vi "Auto Ground Manipulator Command_wrapper.vi"() -> ()   [LabVIEW 2020]
uses:
  <vilib>/Rock Robotics/WPI/Framework/Command Status Info.ctl
  <vilib>/Rock Robotics/WPI/Framework/Completion Status.ctl
  <vilib>/Rock Robotics/WPI/Framework/Completion Notifier.ctl
  intake sub/Implementation/Typedef/intake typedef.ctl
panel:
  out "Command Info Out":T1
  in  "intake modes":T4
  in  "Command Info In":T1
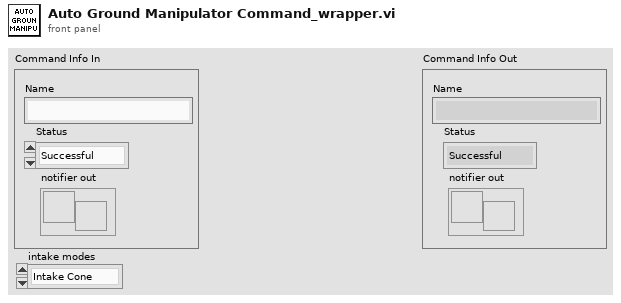
[diagram p1: front panel]
types:
  T1 = typedef "Command Status Info.ctl" = cluster{"Name":string, "Status":T2, "notifier out":T3}
  T2 = typedef "Completion Status.ctl" = enum16{"Successful", "Aborted", "Incomplete"}
  T3 = typedef "Completion Notifier.ctl" = refnum<notifier>
  T4 = typedef "intake typedef.ctl" = enum16{"Intake Cone", "Intake Cube", "Outtake/Score"}
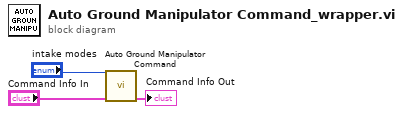
[diagram p0: block diagram]
diagram:
  n1 = call "Auto Ground Manipulator Command.vi"("Command Info In"="Command Info In", "intake modes"="intake modes") -> ("Command Info Out"=→"Command Info Out":T1)  [unwired: 9 in]
